vi "Shutdown FPGA Signals.vi"(8 "error in":errorcluster) -> (0 "error out":errorcluster)   [LabVIEW 2024, in "FPGA Interface.lvlib"]
uses:
  FPGA Interface.lvlib
  FPGA Reference - Get.vi
  <vilib>/Utility/error.llb/Error Cluster From Error Code.vi
  <vilib>/rvi/errors/niLvFpgaAdjustHostInterfaceError.vi
  <vilib>/rvi/interface/nirviReadWriteControl/nirviReadWriteControl.xnode
  Type Definitions/ECU FPGA Reference.ctl
  FPGA Bitfiles/ecu-9030_FPGATarget_FPGAMain_pDLqQGhG1UY.lvbitx
  NiFpgaLv.dll
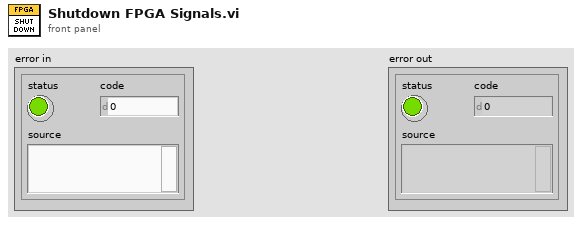
[diagram p1: front panel]
types:
  T1 = typedef "ECU FPGA Reference.ctl" = refnum<k20>
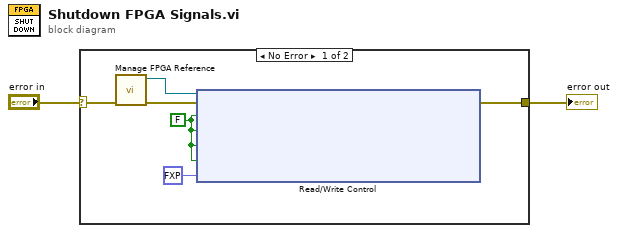
[diagram p0: block diagram]
diagram:
  n1 = case shown="No Error" "error in" {
    selector: "error in" -> [w3 w9]
    tunnel: [w4 w9] -> w2
    frame No Error {
      w5 = FALSE ("DO1")
      n2 = call-poly "Manage FPGA Reference.vi"("error in"=w3) -> ("error out"=w7:errorcluster, "FPGA Reference Out"=w8:T1)  [unwired: 9 in]
      n3 = xnode "Read/Write Control"("FPGA VI Reference In"=w8, "error in"=w7, "DO1"=w5, "DO2"=w5, "Enable PWM"=w5, "Enable Sinewave"=w5, "Voltage Out"=fxp<+/-,20,5> 0.0) -> ("error out"=w4:errorcluster)  [unwired: 1 out]
    }
    frame Error {
    }
  }
  "error out" <- w2
